vi "Get Attributes.vi"(8 "error in (no error)":errorcluster, 11 "For Loop Dialog in":refnum<class "TestStep Edit Dialog.lvclass">) -> (0 "error out":errorcluster, 3 "For Loop Dialog out":refnum<class "TestStep Edit Dialog.lvclass">)   [LabVIEW 2019, in "TestStep Edit Dialog.lvclass"]
uses:
  <vilib>/gpm_packages/@cs/Test-executive-builder/Source/Test Executive Builder Dialogs/TestStep Edit Dialog/TestStep Edit Dialog.lvclass
  C:/Program Files/National Instruments/LabVIEW 2019/vi.lib/gpm_packages/@cs/Test-executive-builder/Source/Test Executive Builder Dialogs/ITest Executive Builder Dialog/ITest Executive Builder Dialog.lvclass
  <vilib>/gpm_packages/@cs/Test-executive-builder/Source/Test Executive Builder Dialogs/ITest Executive Builder Dialog/ITest Executive Builder Dialog.lvclass/ITest Executive Builder Dialog.ctl
  <vilib>/gpm_packages/@cs/Test-executive-builder/Source/Test Executive Builder Dialogs/TestStep Edit Dialog/TestStep Edit Dialog.lvclass/TestStep Edit Dialog.ctl
  191dc990-9661-4c30-b313-8302c425e24e.vi
  bd3c3d9a-c639-4d3a-a825-43e3a07e4ab5.vi
  <vilib>/Utility/error.llb/Clear Errors.vi
  <vilib>/gpm_packages/@cs/test-executive/Source/Test Executive/ITestExecutive/ITest Executive.lvclass
  <vilib>/gpm_packages/@cs/Test-executive-builder/Source/Data Type Handler/Test Executive Builder Data Type Handler.lvclass
  <vilib>/gpm_packages/@cs/Test-executive-builder/Source/Test Executive Builder Dialogs/ITest Executive Builder Dialog/ITest Executive Builder Dialog.lvclass
  <vilib>/gpm_packages/@cs/test-executive/Source/Test Executive/TestExecutive Ref/TestExecutive Ref.lvclass
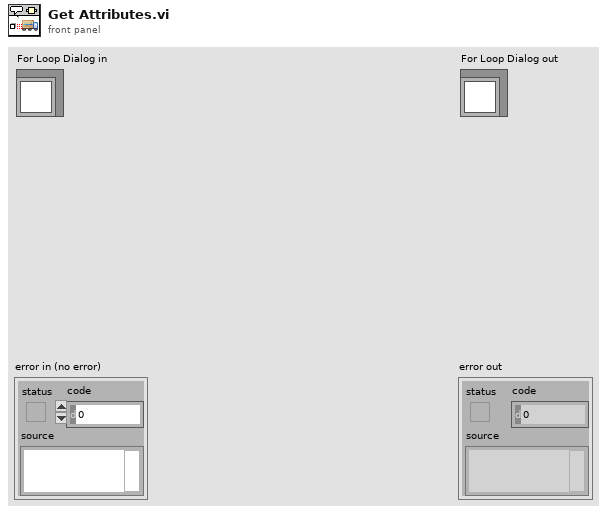
[diagram p1: front panel]
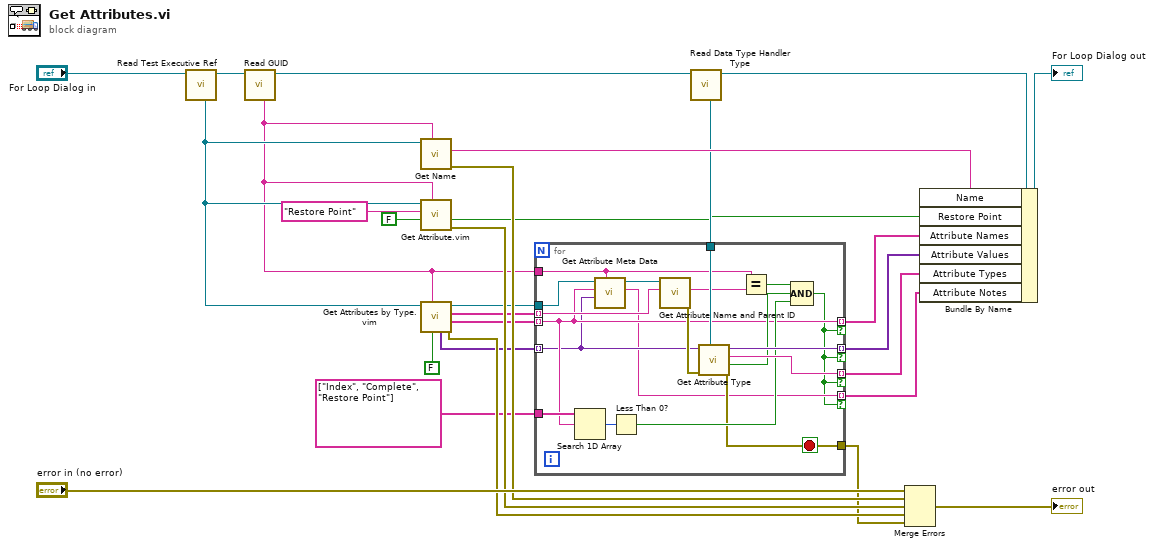
[diagram p0: block diagram]
diagram:
  n1 = call <vilib>:"Read Test Executive Ref.vi"("ITest Executive Builder Dialog in"="For Loop Dialog in") -> ("ITest Executive Builder Dialog out"=w27:refnum<class "TestStep Edit Dialog.lvclass">, "Test Executive Ref"=w18:refnum<data-value>)  [unwired: 9 in]
  n2 = call <vilib>:"Read GUID.vi"("ITest Executive Builder Dialog in"=w27) -> ("ITest Executive Builder Dialog out"=w10:refnum<class "TestStep Edit Dialog.lvclass">, "GUID"=w11:string)  [unwired: 9 in]
  n3 = call <vilib>:"Get Name.vi"("Unique ID"=w11, "Test Executive Ref"=w18) -> ("error out"=w19:errorcluster, "Name"=w26:string)  [unwired: 5 in, 3 out]
  n4 = call "Get Attribute.vim"("ID"=w11, "Type"=FALSE, "Attribute Name"="Restore Point", "Test Executive Ref"=w18) -> ("error out"=w20:errorcluster, "Attribute"=w6:bool)  [unwired: 3 in, 3 out]
  n5 = call "Get Attributes by Type.vim"("Recurse Up List (Default=True)"=FALSE, "ID"=w11, "Test Executive Ref"=w18) -> ("error out"=w17:errorcluster, "Names"=w14:string[], "IDs"=w13:string[], "Test Executive Ref out"=w12:refnum<data-value>, "Attributes"=w15:variant[])  [unwired: 4 in]
  n6 = call <vilib>:"Read Data Type Handler Type.vi"("ITest Executive Builder Dialog in"=w10) -> ("ITest Executive Builder Dialog out"=w9:refnum<class "TestStep Edit Dialog.lvclass">, "Data Type Handler"=w8:refnum<class "Test Executive Builder Data Type Handler.lvclass">)  [unwired: 9 in]
  n7 = for {
    tunnel: w15 -> [w31] mode=indexing
    tunnel: w14 -> [w32] mode=indexing
    tunnel: w13 -> [w47] mode=indexing
    tunnel: w12 -> [w35]
    tunnel: w11 -> [w33]
    tunnel: w8 -> [w46]
    tunnel: [w36] -> w7
    tunnel: [w32] -> w4 mode=indexing if=w29
    tunnel: [w44] -> w2 mode=indexing if=w29
    tunnel: [w41] -> w3 mode=indexing if=w29
    tunnel: string[] ["Index", "Complete", "Restore Point"] -> [w39]
    tunnel: [w30] -> w1 mode=indexing if=w29
    stop <- w36 stop-if-true
    n8 = Search 1D Array(1D array=w39, element=w32) -> (index of element=w38:i32)  [unwired: 1 in]
    n9 = call <vilib>:"Get Attribute Meta Data.vi"("Unique ID"=w33, "Attribute Type"=w31, "Attribute Name"=w32, "Test Executive Ref"=w35) -> ("Meta Data"=w30:string, "Test Executive Ref out"=w34:refnum<data-value>)  [unwired: 4 in, 2 out]
    n10 = Less Than 0?(x=w38) -> (x < 0?=w37:bool)
    n11 = call <vilib>:"Get Attribute Name and Parent ID.vi"("Tag"=w47, "Test Executive Ref"=w34) -> ("error out"=w45:errorcluster, "Parent ID"=w43:string)  [unwired: 6 in, 2 out]
    n12 = call-dynamic "Get Attribute Type.vi"("Test Executive Builder Data Type Handler in"=w46, "error in (no error)"=w45, "Potential Attribute in"=w31) -> ("error out"=w36:errorcluster, "Valid Type?"=w40:bool, "Attribute Type"=w44:string, "Potential Attribute out"=w41:variant)  [unwired: 5 in]
    n13 = Equal?(x=w33, y=w43) -> (x = y?=w42:bool)
    n14 = Compound Arithmetic op=AND(w42, w40, w37) -> (w29:bool)
  }
  n15 = Merge Errors("error in (no error)", w19, w20, w17, w7) -> (→"error out":errorcluster)
  n16 = Bundle By Name(cluster=w9, "Name"=w26, "Restore Point"=w6, "Attribute Names"=w4, "Attribute Values"=w3, "Attribute Types"=w2, "Attribute Notes"=w1) -> (→"For Loop Dialog out":refnum<class "TestStep Edit Dialog.lvclass">)
